vi "OAT Get Vector Reference (1 Channel).vi"(0 "scaled signal [EU]":waveform(dbl)={"t0"=timestamp(0 s since 1904-01-01), "dt"=0.0, "Y"=[]}, 1 "reference output mode":T1(ring), 2 "reset? (F)":bool, 5 "speed profile":T2 {"speed [RPM]" format="%.2f"; "time [s]" format="%.2f"}, 7 "pulse/revolution (1)":i32=1, 9 "orders to compensate (1.0)":dbl[](array[numeric])=[1.0] format="%.2f", 11 "error in (no error)":errorcluster, 12 "bandwidth [order]":dbl=1.0 format="%.2f") -> (4 "vector references":cdb[](array[numeric]) format="%.2f", 15 "error out":errorcluster)   [LabVIEW 2017, in "SoundVib_RefDataProcess.lvlib"]
doc: "Computes the vector references of the specified orders from the slow-roll vibration signals. Use the vector references to compensate shaft bow or runout errors. Wire data to the <B>scaled signal [EU]</B> input to determine the polymorphic instance to use or manually select the instance."
uses:
  <vilib>/addons/Sound and Vibration/Order Analysis/Referece Data Processing/SoundVib_RefDataProcess.lvlib
  <vilib>/addons/Sound and Vibration/Order Analysis/Tach Process/SubVIs/speed profile.ctl
  <vilib>/addons/_NISVFA/_Shared subVIs/Common/svc_Check for Waveform Parameter Continuity (no state).vi
  <vilib>/addons/_NISVFA/_Shared subVIs/Common/svc_Get SV Channel Info.vi
  <vilib>/addons/Sound and Vibration/Order Analysis/Resample Order Tracking/OAT Order Magnitude and Phase (Even Angle Signal, 1 Channel).vi
  <vilib>/addons/Sound and Vibration/Order Analysis/Resample Order Tracking/OAT Convert to Even Angle Signal (1 Channel).vi
  <vilib>/addons/_NISVFA/_Shared subVIs/Common/svc_Engineering Units to Unit Label.vi
  <vilib>/addons/_NISVFA/_Shared subVIs/Common/svc_Unit Label to Engineering Units.vi
  <vilib>/Analysis/NI_AALPro.lvlib
  <vilib>/addons/Sound and Vibration/Order Analysis/Resample Order Tracking/SoundVib_OrderTracking.lvlib
  <vilib>/addons/Sound and Vibration/Order Analysis/Tach Process/SoundVib_TachProcess.lvlib
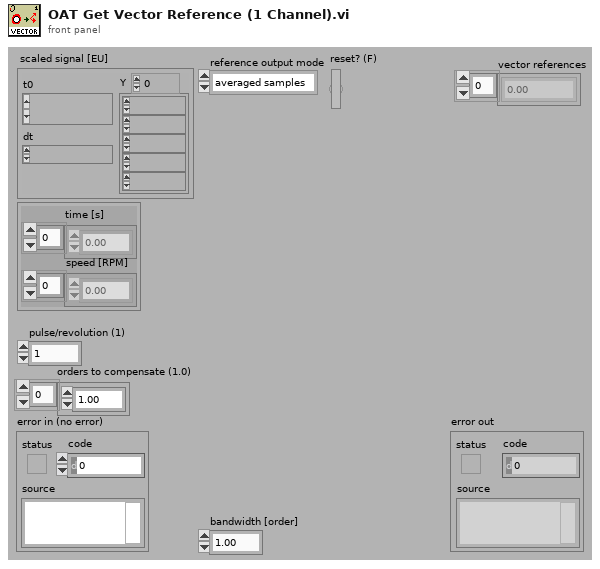
[diagram p1: front panel]
types:
  T1 = enum16{"averaged samples", "initial samples", "final samples"}
  T2 = typedef "SoundVib_TachProcess.lvlib/speed profile.ctl" = cluster{"time [s]":dbl[], "speed [RPM]":dbl[]}
  T3 = cluster{"dt":bool, "t0 continuity":bool, "array length":bool, "channel info":bool, "name":bool}
  T4 = cluster{"dB on? (T)":bool, "unwrap phase? (T)":bool, "unit in degree? (T)":bool}
  T5 = typedef "svc_Resampled Channel Info.ctl" = cluster{"channel name":string, "description":string, " channel info":T6}
  T6 = typedef "svc_Channel Info.ctl" = cluster{"sensor sensitivity":dbl, "engineering units":T7, "dB reference":dbl, "custom label":string, "weighting filter":T8, "pregain":dbl}
  T7 = typedef "svc_Engineering Units Text Ring.ctl" = u16
  T8 = typedef "svc_Weighting Filter Text Ring.ctl" = u16
  T9 = typedef "OAT Position Info.ctl" = cluster{"positions [s]":dbl[], "samples/rev":dbl}
  T10 = cluster{"time/rev/rpm":dbl[], "magnitude":dbl[]}[]
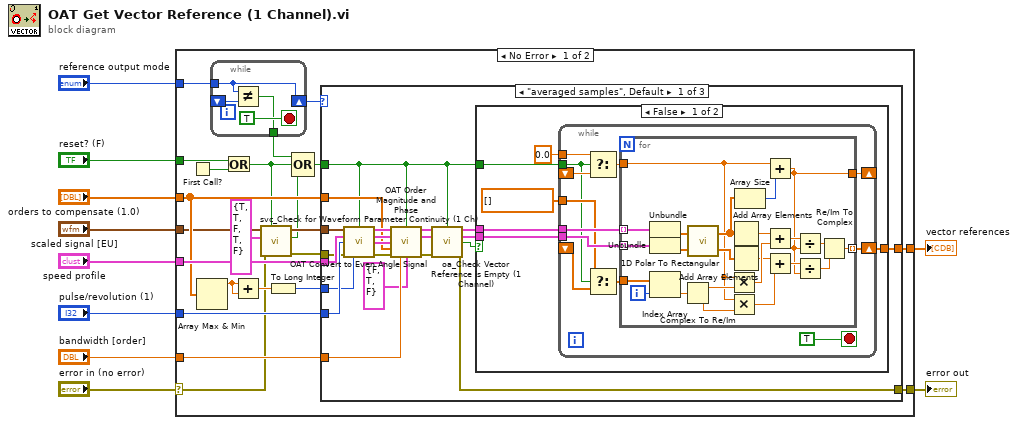
[diagram p0: block diagram]
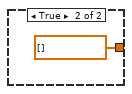
[diagram p2: hidden frame]
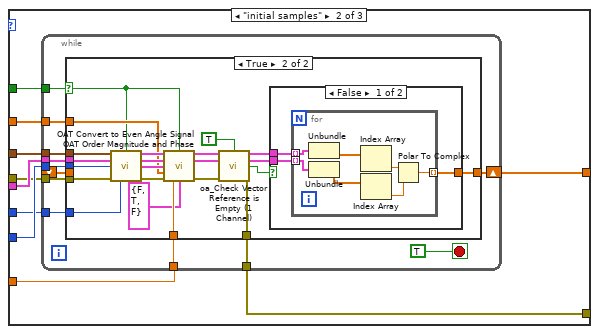
[diagram p3: hidden frame]
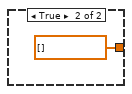
[diagram p5: hidden frame]
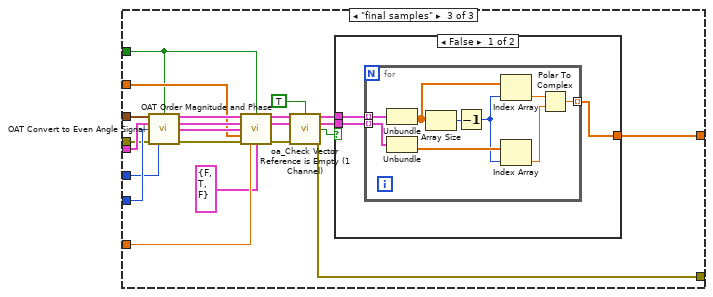
[diagram p6: hidden frame]
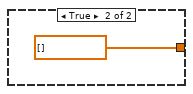
[diagram p7: hidden frame]
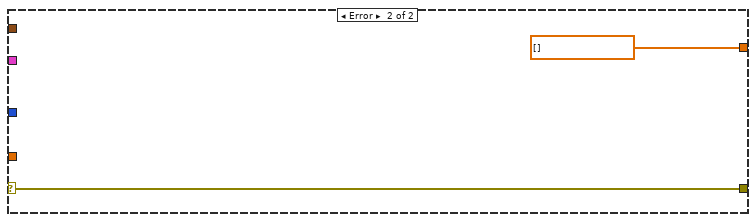
[diagram p8: hidden frame]
diagram:
  n1 = case shown="No Error" "error in (no error)" {
    selector: "error in (no error)" -> [w12 w192]
    tunnel: "scaled signal [EU]" -> [w17 _]
    tunnel: "speed profile" -> [w32 _]
    tunnel: "pulse/revolution (1)" -> [w31 _]
    tunnel: [w30 cdb[] []] -> w6
    tunnel: [w29 w192] -> w5
    tunnel: "bandwidth [order]" -> [w28 _]
    tunnel: "orders to compensate (1.0)" -> [w21 _]
    tunnel: "reference output mode" -> [w27 _]
    tunnel: "reset? (F)" -> [w18 _]
    frame No Error {
      n2 = First Call?() -> (First Call?: T/F=w19:bool)
      n3 = Array Max & Min(array=w21) -> (max value=w22:dbl)  [unwired: 3 out]
      n4 = while {
        shift-right: [w36] -> w26
        shift-left: _ -> [w35]
        tunnel: w27 -> [w36]
        tunnel: [w33] -> w25
        stop <- TRUE stop-if-true
        n5 = Not Equal?(x=w36, y=w35) -> (x != y?=w33:bool)
      }
      n6 = Or(x=w18, y=w19) -> (x .or. y?=w16:bool)
      n7 = Add(x=w22, y=w22) -> (x+y=w23:dbl)
      n8 = call <vilib>:"svc_Check for Waveform Parameter Continuity (1 Ch).vi"("restart averaging (F)"=w16, "error in (no error)"=w12, "checks for channel parameter change"=T3 {"dt"=TRUE, "t0 continuity"=TRUE, "array length"=FALSE, "channel info"=TRUE, "name"=FALSE}, "scaled signal [EU]"=w17) -> ("error out"=w11:errorcluster, "waveform parameter changed"=w13:bool, "dup scaled signal [EU]"=w15:waveform(dbl))  [unwired: 2 in, 3 out]
      n9 = To Long Integer(number=w23) -> (32bit integer=w20:i32)
      n10 = Compound Arithmetic op=OR(w25, w16, w13) -> (w24:bool)
      n11 = case shown="\"averaged samples\", Default" w26 {
        tunnel: w15 -> [w57 w109 w178]
        tunnel: w32 -> [w56 w108 w177]
        tunnel: w31 -> [w55 w107 w176]
        tunnel: w11 -> [w54 w106 w175]
        tunnel: [w48 w105 w174] -> w30
        tunnel: [w39 w104 w160] -> w29
        tunnel: w28 -> [w49 w103 w173]
        tunnel: w21 -> [w47 w102 w168]
        tunnel: w24 -> [w37 w101 w158]
        tunnel: w20 -> [w46 w100 w167]
        frame "averaged samples", Default {
          n12 = call-poly <vilib>:"OAT Convert to Even Angle Signal.vi"("scaled signal [EU]"=w57, "reset? (F)"=w37, "speed profile"=w56, "pulse/revolution (1)"=w55, "error in (no error)"=w54, "max order (auto)"=w46) -> ("even-angle signal"=w53:cluster{"r0":dbl, "dr":dbl, "Y":dbl[]}, "even-angle channel info"=w52:T5, "even-angle position info"=w51:T9, "error out"=w50:errorcluster)  [unwired: 5 in, 1 out]
          n13 = call-poly <vilib>:"OAT Order Magnitude and Phase.vi"("even-angle signal"=w53, "reset? (F)"=w37, "even-angle channel info"=w52, "even-angle position info"=w51, "orders to compute (1.0)"=w47, "error in (no error)"=w50, "bandwidth [order]"=w49, "view"=T4 {"dB on? (T)"=FALSE, "unwrap phase? (T)"=TRUE, "unit in degree? (T)"=FALSE}) -> ("magnitudes [RMS]"=w44:T10, "phases [phase lag]"=w42:cluster{"time/rev/rpm":dbl[], "phase":dbl[]}[], "error out"=w40:errorcluster)  [unwired: 2 in, 3 out]
          n14 = call <vilib>:"oa_Check Vector Reference is Empty (1 Channel).vi"("magnitudes [RMS] in"=w44, "reset? (F)"=w37, "phases [phase lag] in"=w42, "error in (no error)"=w40) -> ("magnitudes [RMS] out"=w43:T10, "phases [phase lag] out"=w41:cluster{"time/rev/rpm":dbl[], "phase":dbl[]}[], "empty?"=w38:bool, "error out"=w39:errorcluster)  [unwired: 8 in]
          n15 = case shown="False" w38 {
            tunnel: [w63 cdb[] []] -> w48
            tunnel: w37 -> [w60 _]
            tunnel: w43 -> [w59 _]
            tunnel: w41 -> [w58 _]
            frame False {
              n16 = while {
                tunnel: w59 -> [w75]
                tunnel: w58 -> [w74]
                shift-right: [w71] -> _
                shift-left: _ -> [w70]
                shift-right: [w72] -> w63
                shift-left: _ -> [w68]
                tunnel: w60 -> [w65]
                tunnel: 0.0 -> [w67]
                tunnel: cdb[] [] -> [w66]
                stop <- TRUE stop-if-true
                n17 = Select(t=w67, s=w65, f=w70) -> (s? t:f=w69:dbl)
                n18 = Select(t=w66, s=w65, f=w68) -> (s? t:f=w64:cdb[])
                n19 = for {
                  tunnel: w75 -> [w98] mode=indexing
                  tunnel: w74 -> [w97] mode=indexing
                  tunnel: [w95] -> w72 mode=indexing
                  tunnel: [w82] -> w71
                  tunnel: w69 -> [w76]
                  tunnel: w64 -> [w79]
                  i -> [w77]
                  n20 = Unbundle(w98) -> ("magnitude"=w96:dbl[])  [unwired: 1 out]
                  n21 = Unbundle(w97) -> ("phase"=w94:dbl[])  [unwired: 1 out]
                  n22 = Index Array(array=w79, index=w77) -> (element=w78:cdb)
                  n23 = Complex To Re/Im(x + iy=w78) -> (x=w92:dbl, y=w91:dbl)
                  n24 = call <vilib>:"1D Polar To Rectangular.vi"("Magnitude"=w96, "Phase"=w94) -> ("X"=w90:dbl[], "Y"=w89:dbl[])  [unwired: 1 out]
                  n25 = Multiply(x=w76, y=w92) -> (x*y=w87:dbl)
                  n26 = Multiply(x=w76, y=w91) -> (x*y=w85:dbl)
                  n27 = Add Array Elements(numeric array=w90) -> (sum=w88:dbl)
                  n28 = Add Array Elements(numeric array=w89) -> (sum=w86:dbl)
                  n29 = Array Size(array=w90) -> (size(s)=w93:i32)
                  n30 = Add(x=w76, y=w93) -> (x+y=w82:dbl)
                  n31 = Add(x=w88, y=w87) -> (x+y=w84:dbl)
                  n32 = Add(x=w86, y=w85) -> (x+y=w83:dbl)
                  n33 = Divide(x=w84, y=w82) -> (x/y=w81:dbl)
                  n34 = Divide(x=w83, y=w82) -> (x/y=w80:dbl)
                  n35 = Re/Im To Complex(1:w80, 2:w81) -> (0:w95:cdb)
                }
              }
            }
            frame True {
            }
          }
        }
        frame "initial samples" {
          n36 = while {
            tunnel: w109 -> [w121]
            tunnel: w108 -> [w120]
            tunnel: w107 -> [w119]
            tunnel: w106 -> [w118]
            tunnel: [w116] -> w104
            tunnel: w103 -> [w115]
            tunnel: w102 -> [w111]
            tunnel: w101 -> [w114]
            shift-right: [w117] -> w105
            shift-left: _ -> [w112]
            tunnel: w100 -> [w110]
            stop <- TRUE stop-if-true
            n37 = case shown="True" w114 {
              selector: w114 -> [_ w125]
              tunnel: w121 -> [_ w145]
              tunnel: w120 -> [_ w144]
              tunnel: w119 -> [_ w143]
              tunnel: w118 -> [w123 w142]
              tunnel: [w122 w137] -> w117
              tunnel: [w123 w127] -> w116
              tunnel: w115 -> [_ w136]
              tunnel: w112 -> [w122 _]
              tunnel: w111 -> [_ w135]
              tunnel: w110 -> [_ w134]
              frame False {
              }
              frame True {
                n38 = call-poly <vilib>:"OAT Convert to Even Angle Signal.vi"("scaled signal [EU]"=w145, "reset? (F)"=w125, "speed profile"=w144, "pulse/revolution (1)"=w143, "error in (no error)"=w142, "max order (auto)"=w134) -> ("even-angle signal"=w141:cluster{"r0":dbl, "dr":dbl, "Y":dbl[]}, "even-angle channel info"=w140:T5, "even-angle position info"=w139:T9, "error out"=w138:errorcluster)  [unwired: 5 in, 1 out]
                n39 = call-poly <vilib>:"OAT Order Magnitude and Phase.vi"("even-angle signal"=w141, "reset? (F)"=w125, "even-angle channel info"=w140, "even-angle position info"=w139, "orders to compute (1.0)"=w135, "error in (no error)"=w138, "bandwidth [order]"=w136, "view"=T4 {"dB on? (T)"=FALSE, "unwrap phase? (T)"=TRUE, "unit in degree? (T)"=FALSE}) -> ("magnitudes [RMS]"=w132:T10, "phases [phase lag]"=w130:cluster{"time/rev/rpm":dbl[], "phase":dbl[]}[], "error out"=w128:errorcluster)  [unwired: 2 in, 3 out]
                n40 = call <vilib>:"oa_Check Vector Reference is Empty (1 Channel).vi"("magnitudes [RMS] in"=w132, "reset? (F)"=TRUE, "phases [phase lag] in"=w130, "error in (no error)"=w128) -> ("magnitudes [RMS] out"=w131:T10, "phases [phase lag] out"=w129:cluster{"time/rev/rpm":dbl[], "phase":dbl[]}[], "empty?"=w126:bool, "error out"=w127:errorcluster)  [unwired: 8 in]
                n41 = case shown="False" w126 {
                  tunnel: [w148 cdb[] []] -> w137
                  tunnel: w131 -> [w147 _]
                  tunnel: w129 -> [w146 _]
                  frame False {
                    n42 = for {
                      tunnel: w147 -> [w155] mode=indexing
                      tunnel: w146 -> [w154] mode=indexing
                      tunnel: [w149] -> w148 mode=indexing
                      n43 = Unbundle(w155) -> ("magnitude"=w153:dbl[])  [unwired: 1 out]
                      n44 = Unbundle(w154) -> ("phase"=w152:dbl[])  [unwired: 1 out]
                      n45 = Index Array(array=w153) -> (element=w151:dbl)  [unwired: 1 in]
                      n46 = Index Array(array=w152) -> (element=w150:dbl)  [unwired: 1 in]
                      n47 = Polar To Complex(1:w150, 2:w151) -> (0:w149:cdb)
                    }
                  }
                  frame True {
                  }
                }
              }
            }
          }
        }
        frame "final samples" {
          n48 = call-poly <vilib>:"OAT Convert to Even Angle Signal.vi"("scaled signal [EU]"=w178, "reset? (F)"=w158, "speed profile"=w177, "pulse/revolution (1)"=w176, "error in (no error)"=w175, "max order (auto)"=w167) -> ("even-angle signal"=w172:cluster{"r0":dbl, "dr":dbl, "Y":dbl[]}, "even-angle channel info"=w171:T5, "even-angle position info"=w170:T9, "error out"=w169:errorcluster)  [unwired: 5 in, 1 out]
          n49 = call-poly <vilib>:"OAT Order Magnitude and Phase.vi"("even-angle signal"=w172, "reset? (F)"=w158, "even-angle channel info"=w171, "even-angle position info"=w170, "orders to compute (1.0)"=w168, "error in (no error)"=w169, "bandwidth [order]"=w173, "view"=T4 {"dB on? (T)"=FALSE, "unwrap phase? (T)"=TRUE, "unit in degree? (T)"=FALSE}) -> ("magnitudes [RMS]"=w165:T10, "phases [phase lag]"=w163:cluster{"time/rev/rpm":dbl[], "phase":dbl[]}[], "error out"=w161:errorcluster)  [unwired: 2 in, 3 out]
          n50 = call <vilib>:"oa_Check Vector Reference is Empty (1 Channel).vi"("magnitudes [RMS] in"=w165, "reset? (F)"=TRUE, "phases [phase lag] in"=w163, "error in (no error)"=w161) -> ("magnitudes [RMS] out"=w164:T10, "phases [phase lag] out"=w162:cluster{"time/rev/rpm":dbl[], "phase":dbl[]}[], "empty?"=w159:bool, "error out"=w160:errorcluster)  [unwired: 8 in]
          n51 = case shown="False" w159 {
            tunnel: [w181 cdb[] []] -> w174
            tunnel: w164 -> [w180 _]
            tunnel: w162 -> [w179 _]
            frame False {
              n52 = for {
                tunnel: w180 -> [w190] mode=indexing
                tunnel: w179 -> [w189] mode=indexing
                tunnel: [w185] -> w181 mode=indexing
                n53 = Unbundle(w190) -> ("magnitude"=w184:dbl[])  [unwired: 1 out]
                n54 = Unbundle(w189) -> ("phase"=w188:dbl[])  [unwired: 1 out]
                n55 = Array Size(array=w184) -> (size(s)=w183:i32)
                n56 = Decrement(x=w183) -> (x-1=w182:i32)
                n57 = Index Array(array=w184, index=w182) -> (element=w187:dbl)
                n58 = Index Array(array=w188, index=w182) -> (element=w186:dbl)
                n59 = Polar To Complex(1:w186, 2:w187) -> (0:w185:cdb)
              }
            }
            frame True {
            }
          }
        }
      }
    }
    frame Error {
    }
  }
  "error out" <- w5
  "vector references" <- w6
